vi "Logger Stopped.vi"(8 "error in (no error)":errorcluster, 10 "Logger Stopped":T1, 11 "Log Manager Module in":refnum<class "Log Manager Module.lvclass">) -> (0 "error out":errorcluster, 3 "Log Manager Module out":refnum<class "Log Manager Module.lvclass">)   [LabVIEW 2020, in "VolatusData.lvlib" / "Log Manager Module.lvclass"]
uses:
  Log Manager Module.lvclass
  C:/dev/lv20CE/relink/lv-volatus/Volatus/Module/Module.lvclass
  Logger Stopped.ctl
  Log Manager Module.lvclass/Log Manager Module.ctl
  Logger State.ctl
  Volatus/Event Level.ctl
  Volatus/Module/Module.lvclass/Module.ctl
  Volatus/Module/Module.lvclass
  VolatusData.lvlib
  Volatus/Volatus.lvlib
  C:/dev/lv20CE/relink/lv-volatus/VolatusData/Log Manager Module/Log Manager Module.lvclass
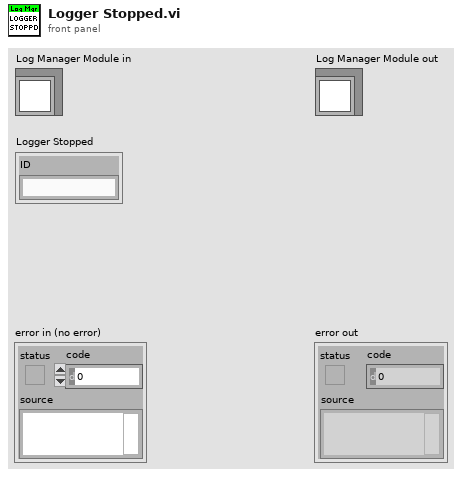
[diagram p1: front panel]
types:
  T1 = typedef "VolatusData.lvlib/Logger Stopped.ctl" = cluster{"ID":string}
  T2 = typedef "VolatusData.lvlib/Logger State.ctl" = enum16{"Unknown", "Idle", "Preparing", "Ready", "Logging", "Stopping"}
  T3 = typedef "VolatusData.lvlib/Log Manager Module.lvclass/Logger.ctl" = cluster{"ID":string, "MsgQ":refnum<class "MessageQ.lvclass">, "State":T2}
  T4 = typedef "Volatus.lvlib/Event Level.ctl" = enum16{"Debug", "Info", "Warning", "Error"}
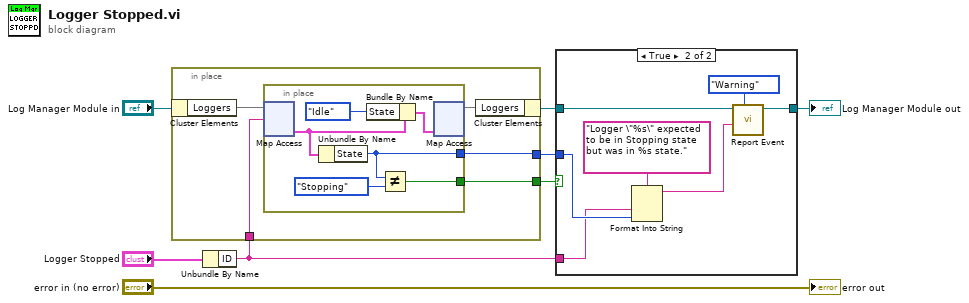
[diagram p0: block diagram]
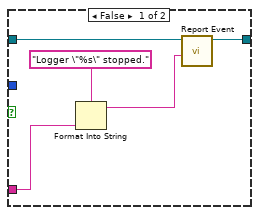
[diagram p2: hidden frame]
diagram:
  n1 = Unbundle By Name("Logger Stopped") -> ("ID"=w1:string)
  n2 = in-place {
    in-place-border: w1 -> [w12]
    in-place-border: [w10] -> w3
    in-place-border: [w9] -> w2
    n3 = in-place-cluster #1("Log Manager Module in") -> ("Loggers"=w13:map{string, T3})
    n4 = in-place {
      in-place-border: [w15] -> w10
      in-place-border: [w14] -> w9
      n5 = in-place-map #2(w13, w12) -> (w17:T3)  [unwired: 1 in, 1 out]
      n6 = Unbundle By Name(w17) -> ("State"=w14:T2)
      n7 = Bundle By Name(cluster=w17, "State"=Logger_State."Idle") -> (w18:T3)
      n8 = Not Equal?(x=w14, y=Logger_State."Stopping") -> (x != y?=w15:bool)
      n9 = in-place-map #2(w18) -> (w11:map{string, T3})  [unwired: 1 in, 2 out]
    }
    n10 = in-place-cluster #1("Loggers"=w11) -> (w5:refnum<class "Log Manager Module.lvclass">)
  }
  n11 = case shown="True" w3 {
    tunnel: w5 -> [w24 w31]
    tunnel: [w23 w29] -> w4
    tunnel: w2 -> [_ w27]
    tunnel: w1 -> [w21 w26]
    frame False {
      n12 = Format Into String(format string="Logger \"%s\" stopped.", w21) -> (resulting string=w20:string)  [unwired: 2 in, 1 out]
      n13 = call "Report Event.vi"("Message"=w20, "Module in"=w24) -> ("Module out"=w23:refnum<class "Log Manager Module.lvclass">)  [unwired: 8 in, 1 out]
    }
    frame True {
      n14 = Format Into String(format string="Logger \"%s\" expected to be in Stopping state but was in %s state.", w26, w27) -> (resulting string=w25:string)  [unwired: 2 in, 1 out]
      n15 = call "Report Event.vi"("Level (Info)"=Event_Level."Warning", "Message"=w25, "Module in"=w31) -> ("Module out"=w29:refnum<class "Log Manager Module.lvclass">)  [unwired: 7 in, 1 out]
    }
  }
  "Log Manager Module out" <- w4
  "error out" <- "error in (no error)"
